vi "VMI Tomography.vi"() -> ()   [LabVIEW 2019]
uses:
  <vilib>/vision/NI_Vision_Development_Module.lvlib
panel:
  in  "CONTROL QWP":refnum<k7>(container)
  in  "Tab Control":enum32{"Setup & Align", "Acquire - Tomography"}(tab)
  out "Counts per Laser Shot :":dbl format="%#.1g"
  in  "Image Size (pixels) :":dbl=400.0
  in  "?":bool
  in  "Acquiring :":bool
  in  "Save?":bool
  in  "Mask Width (pixels) :":dbl
  in  "Mask Centre :":bool
  in  "Threshold Level (%) :":dbl
  in  "Image Centre (x,y) : 2":dbl=223.0
  in  "Image Centre (x,y) :":dbl=312.0
  in  "Symmetrise L/R :":bool
  in  "Symmetrise U/D :":bool
  in  "Centroiding :":bool
  out "Test View":dbl[][](graph)
  out "Integrated Signal Graph":dbl[](graph)
  out "Live Camera View":dbl[][](graph)
  in  "QWP Zero Position :":dbl=174.0
  out "Current Scan :":dbl
  out "Current Angle :":dbl
  out "Current Frame :":i32
  in  "Frames per Scan :":dbl=100.0
  out "Current Image":dbl[][](graph)
  in  "?":refnum<k7>(container)
  in  "Molecule :":string="a_pinene"
  in  "OK Button 2":bool
  in  "HWP Zero Position :":dbl=25.7
  in  "HWP Step Size :":dbl=15.0
  in  "No. of Scans :":dbl=1.0
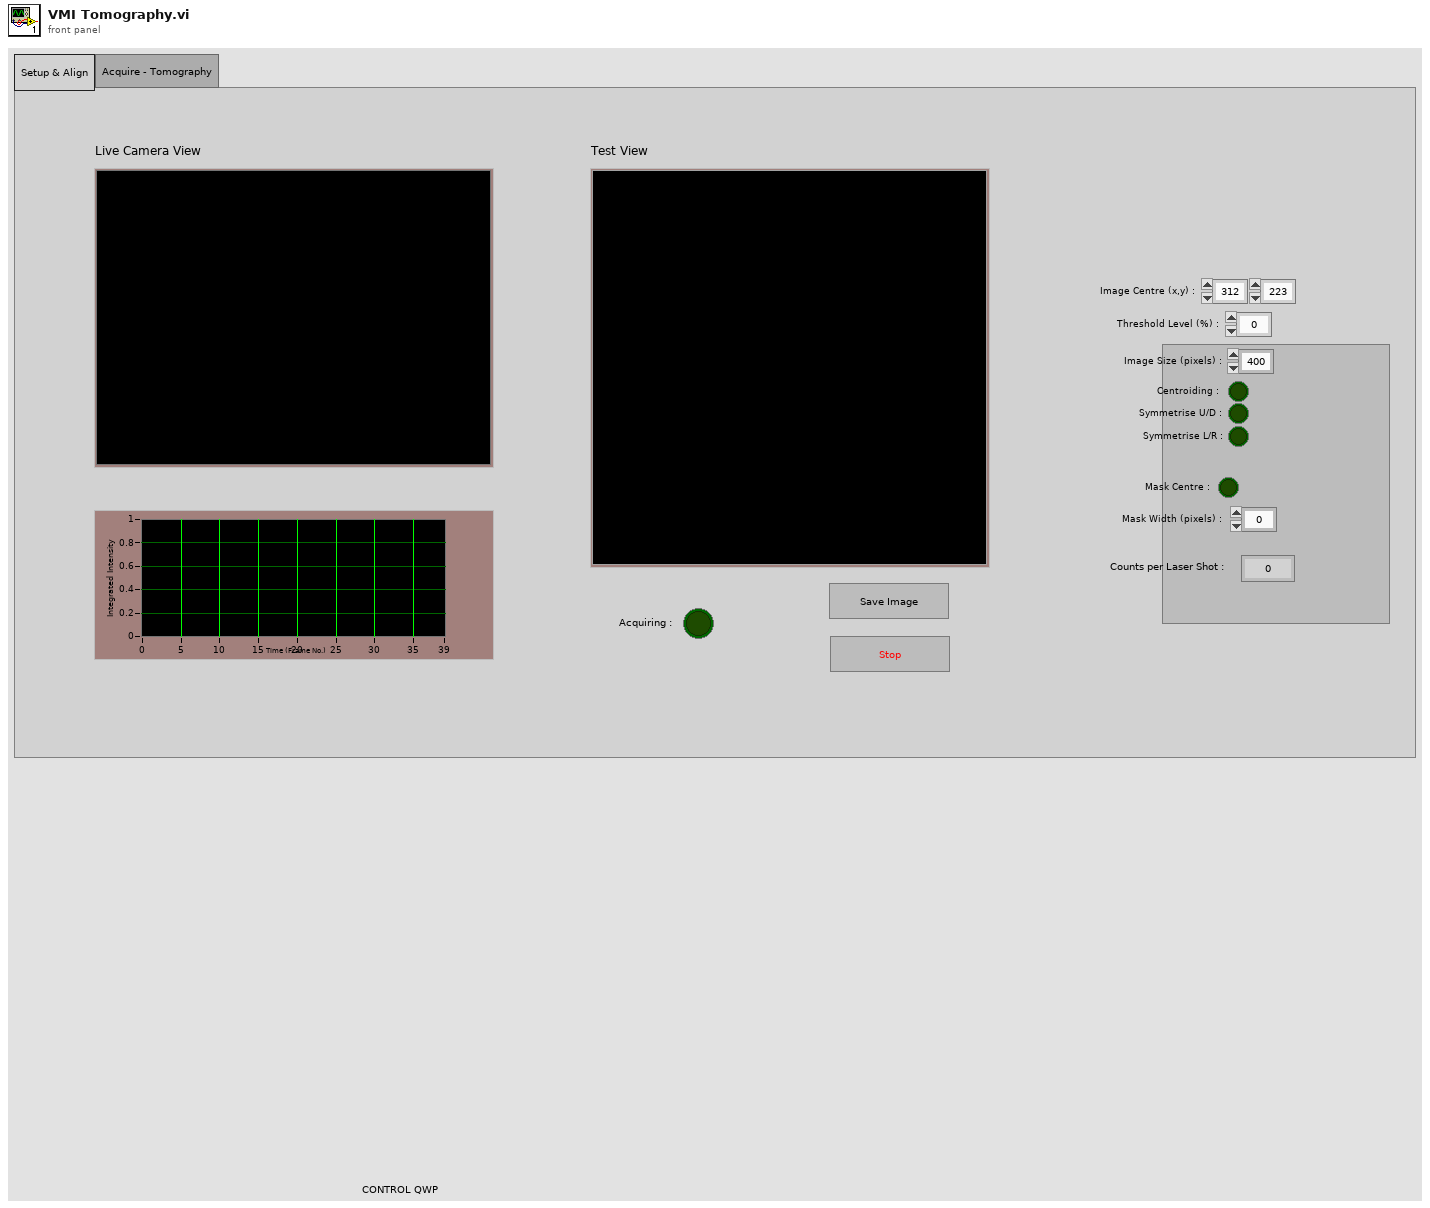
[diagram p1: front panel]
types:
  T1 = typedef "Image Type" = u32
  T2 = typedef "IMAQ Image.ctl" = refnum<image>
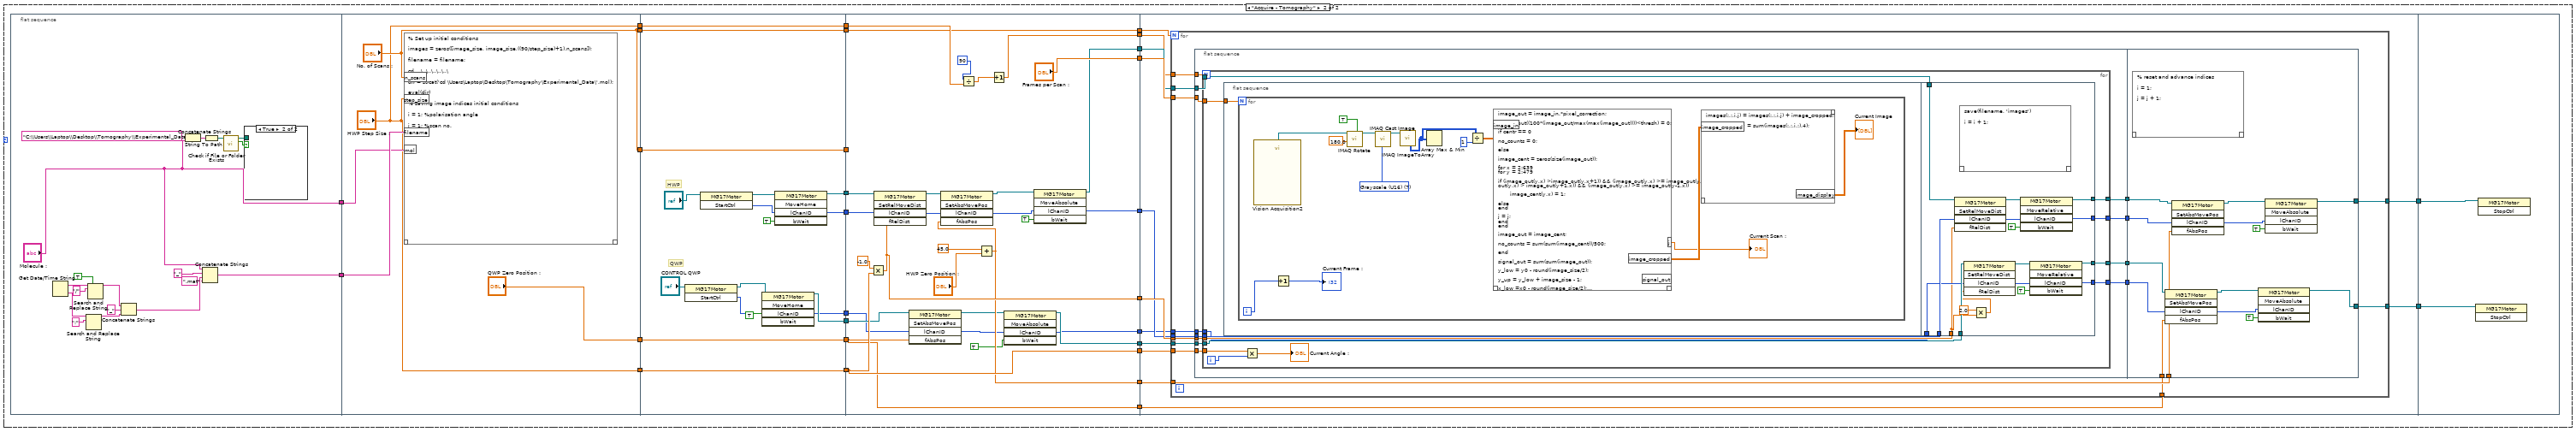
[diagram p3: hidden frame]
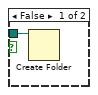
[diagram p4: hidden frame]
diagram:
  n1 = case shown="\"Setup & Align\", Default" "Tab Control" {
    frame "Setup & Align", Default {
      n2 = while {
        i -> [w4]
        stop <- "?" stop-if-true
        n3 = flat-sequence {
          tunnel: [w9] -> w8
          tunnel: w8 -> [w37]
          tunnel: [w36] -> w7
          tunnel: [w35] -> w5
          tunnel: [w31] -> w3
          tunnel: [w18] -> w2
          tunnel: w7 -> [w44]
          tunnel: w5 -> [w40]
          tunnel: w4 -> [_]
          tunnel: w3 -> [w41]
          tunnel: w2 -> [w38]
          frame #0 {
            n4 = script code="% Set up initial variables and define hot pixels\n\npixel_correction = ones(480,640);\n\npixel_correction(445,233) = 0;\npixel_correction(444,232) = 0\npixel_correction(240,208) = 0;\npixel_correction(268,295) = 0;\npixel_correction(440,333) = 0;\npixel_correction(257,482) = 0;\npixel_correction(128,286) = 0;\npixel_correction(208,240) = 0;\npixel_correction(404,604) = 0;\n\npixel_correction(270,304) = 0;\npixel_correction(346,358) = 0;\npixel_correction(220,79) = 0;\npixel_correction(79,218) = 0;\npixel_correction(96,220) = 0;\n\npixel_correction(218,96) = 0;\npixel_correction(268,304) = 0;\npixel_correction(218,79) = 0;\npixel_correction(268,304) = 0;\n\ncd ..\\..\\..\\..\\..\\..\\..\\Users\\Laptop\\Desktop"() -> ()  [unwired: 1 in, 1 out]
          }
          frame #1 {
            w17 = T1 7 items=["Grayscale (U8)", "Grayscale (I16)", "Grayscale (SGL)", "Complex (CSG)", "RGB (U32)", "HSL (U32)", "RGB (U64)", "Grayscale (U16)"] ("Image Type")
            n5 = call "Vision Acquisition"() -> ("Image Out"=w11:T2)  [unwired: 26 in, 1 out]
            n6 = call "IMAQ Rotate"("Maintain Size"=TRUE, "Angle (degrees)"=sgl 180.0, "Image Src"=w11) -> ("Image Dst Out"=w14:T2)  [unwired: 7 in, 1 out]
            n7 = call "IMAQ Cast Image"("Image Type"=w17, "Image Src"=w14) -> ("Image Dst Out"=w16:T2)  [unwired: 8 in, 1 out]
            n8 = call "IMAQ ImageToArray"("Image"=w16) -> ("Image Pixels (U16)"=w15:u16[][])  [unwired: 3 in, 4 out]
            n9 = Array Max & Min(array=w15) -> ()  [unwired: 4 out]
            n10 = Divide(x=w15, y=1) -> (x/y=w9:dbl[][])
          }
          frame #2 {
            n11 = Boolean To (0,1)(Boolean="Mask Centre :") -> (0, 1=w22:i16)
            n12 = Boolean To (0,1)(Boolean="Acquiring :") -> (0, 1=w25:i16)
            n13 = Boolean To (0,1)(Boolean="Symmetrise U/D :") -> (0, 1=w26:i16)
            n14 = Boolean To (0,1)(Boolean="Symmetrise L/R :") -> (0, 1=w29:i16)
            n15 = Boolean To (0,1)(Boolean="Centroiding :") -> (0, 1=w19:i16)
            n16 = script code="image_out = image_in.*pixel_correction;\n\nimage_out((100*(image_out/max(max(image_out))))<thresh) = 0;\n\nif centr == 0\n\nno_counts = 0;\n\nelse\n\nimage_cent = zeros(size(image_out));\n\nfor x = 2:639\nfor y = 2:479\n\nif (image_out(y,x) >image_out(y,x+1)) && (image_out(y,x) >= image_out(y,x-1)) && (image_out(y,x) > image_out(y+1,x)) && (image_out(y,x) >= image_out(y-1,x))\n\n       image_cent(y,x) = 1;\n\nelse\nend\n\nend\nend\n\nimage_out = image_cent;\n\nno_counts = sum(sum(image_cent))/500;\n\nend\n\nsignal_out = sum(sum(image_out));\n\ny_low = y0 - round(image_size/2);\n\ny_up = y_low + image_size - 1;\n\nx_low =x0 - round(image_size/2);\n\nx_up = x_low + image_size - 1;\n\nif acqu == 0\n\n     image_cropped = zeros(image_size);\n\nend\n\nimage_cropped = image_out(y_low:y_up,x_low:x_up) + image_cropped;\n\nif LR == 1\n\n     image_cropped = 0.5*(image_cropped + fliplr(image_cropped));\n\nend\n\nif UD == 1\n\n     image_cropped = 0.5*(image_cropped + flipud(image_cropped));\n\nend\n\nif mask == 1\n\n     x = linspace(-(round(image_size/2)), round(image_size/2), image_size);\n\n     [X, Y] = meshgrid(x,x);\n\n     R = sqrt(X.^2 + Y.^2);\n\n     mask_ = ones(size(R));\n\n     mask_(R<mask_width) = 0;\n\n     image_cropped = image_cropped.*mask_;\n\nend\n\nrange = 1:image_size;\n\ny_int = sum(image_cropped,1);\ny_int = y_int/max(y_int);\n\nx_int = sum(image_cropped,2);\nx_int = x_int/max(x_int);"("image_in"=w37, "image_size"="Image Size (pixels) :", "x0"="Image Centre (x,y) :", "y0"="Image Centre (x,y) : 2", "thresh"="Threshold Level (%) :", "LR"=w29, "UD"=w26, "acqu"=w25, "mask"=w22, "mask_width"="Mask Width (pixels) :", "centr"=w19) -> ("image_out"=w36:dbl[][], "signal_out"=w35:dbl, "image_cropped"=w31:dbl[][], "no_counts"=w18:dbl)  [unwired: 1 in, 4 out]
          }
          frame #3 {
            n17 = feedback #1() -> (w39:dbl[])  [unwired: 1 in]
            n18 = Build Array (concatenate)(w39, w40) -> (w48:dbl[])
            n19 = feedback-in #1(w48) -> ()
            n20 = Array Max & Min(array=w44) -> (max value=w45:dbl)  [unwired: 3 out]
            n21 = Array Max & Min(array=w41) -> (max value=w43:dbl)  [unwired: 3 out]
            n22 = Array Max & Min(array=w48) -> (max value=w47:dbl)  [unwired: 3 out]
            n23 = Divide(x=w44, y=w45) -> (x/y=→"Live Camera View":dbl[][])
            n24 = Divide(x=w41, y=w43) -> (x/y=→"Test View":dbl[][])
            n25 = Divide(x=w48, y=w47) -> (x/y=→"Integrated Signal Graph":dbl[])
            "Counts per Laser Shot :" <- w38
          }
          frame #4 {
            n26 = case shown="True" "Save?" {
              frame False {
              }
              frame True {
                n27 = script code="image = image_cropped;\n\nuisave('image','image.mat')"() -> ()  [unwired: 1 in, 1 out]
              }
            }
          }
        }
      }
    }
    frame "Acquire - Tomography" {
      n28 = flat-sequence {
        tunnel: [w81] -> w73
        tunnel: ["Molecule :"] -> w72
        tunnel: ["No. of Scans :"] -> w76
        tunnel: ["HWP Step Size :"] -> w74
        tunnel: w73 -> [w103]
        tunnel: w72 -> [w102]
        tunnel: ["No. of Scans :"] -> w71
        tunnel: ["HWP Step Size :"] -> w64
        tunnel: ["QWP Zero Position :"] -> w56
        tunnel: [w116] -> w79
        tunnel: [w115] -> w78
        tunnel: [w114] -> w77
        tunnel: w76 -> [w114]
        tunnel: [w113] -> w75
        tunnel: w74 -> [w113]
        tunnel: w71 -> [w112]
        tunnel: [w112] -> w70
        tunnel: [w111] -> w65
        tunnel: w64 -> [w111]
        tunnel: [w106] -> w58
        tunnel: [w105] -> w57
        tunnel: w56 -> [w104]
        tunnel: [w104] -> w55
        tunnel: w79 -> [w149]
        tunnel: w78 -> [w148]
        tunnel: w77 -> [w129]
        tunnel: w75 -> [w131]
        tunnel: w70 -> [_]
        tunnel: ["Frames per Scan :"] -> w69
        tunnel: [w138] -> w68
        tunnel: [w137] -> w67
        tunnel: [w136] -> w66
        tunnel: w65 -> [w135]
        tunnel: [w132] -> w63
        tunnel: [w131] -> w62
        tunnel: [w130] -> w61
        tunnel: [w129] -> w60
        tunnel: w58 -> [w125]
        tunnel: w57 -> [w124]
        tunnel: w55 -> [w121]
        tunnel: [w123] -> w54
        tunnel: [w122] -> w53
        tunnel: [w121] -> w51
        tunnel: w69 -> [w162]
        tunnel: w68 -> [w161]
        tunnel: w67 -> [w160]
        tunnel: w66 -> [w159]
        tunnel: w63 -> [w158]
        tunnel: w62 -> [w157]
        tunnel: w61 -> [w156]
        tunnel: w60 -> [w155]
        tunnel: [w154] -> w59
        tunnel: w54 -> [w153]
        tunnel: w53 -> [w152]
        tunnel: [w151] -> w52
        tunnel: w51 -> [w150]
        tunnel: w59 -> [w251]
        tunnel: w52 -> [w250]
        frame #0 {
          n29 = Get Date/Time String() -> (date string=w92:string, time string=w89:string)  [unwired: 3 in]
          n30 = Search and Replace String(input string=w89, search string=":") -> (result string=w86:string)  [unwired: 6 in, 3 out]
          n31 = Search and Replace String(replace all?=TRUE ("replace all? (F)"), input string=w92, search string="/") -> (result string=w87:string)  [unwired: 5 in, 3 out]
          n32 = Concatenate Strings(w87, "_" ("string"), w86) -> (w83:string)
          n33 = Concatenate Strings("C:\\Users\\Laptop\\Desktop\\Tomography\\Experimental_Data\\", "Molecule :") -> (w93:string)
          n34 = Concatenate Strings("Molecule :", "_" ("string"), w83, ".mat" ("string")) -> (w81:string)
          n35 = String To Path(string=w93) -> (path=w96:path)
          n36 = call <vilib>:"Check if File or Folder Exists.vi"("path"=w96) -> ("file or folder exists?"=w95:bool, "dup path"=w94:path)  [unwired: 8 in, 1 out]
          n37 = case shown="True" w95 {
            tunnel: w94 -> [w98 _]
            frame False {
              n38 = Create Folder(path (use dialog)=w98) -> ()  [unwired: 2 in, 3 out]
            }
            frame True {
            }
          }
        }
        frame #1 {
          n39 = script code="% Set up initial conditions\n\nimages = zeros([image_size, image_size,((90/step_size)+1),n_scans]);\n\nfilename = filename;\n\ncd  ..\\..\\..\\..\\..\\..\\\n\ndir = strcat('cd \\Users\\Laptop\\Desktop\\Tomography\\Experimental_Data\\',mol);\n\neval(dir)\n\n% saving image indices initial conditions\n\ni = 1; %polarisation angle\n\nj = 1; %scan no."("n_scans"="No. of Scans :", "step_size"="HWP Step Size :", "filename"=w103, "mol"=w102) -> ()  [unwired: 1 in, 1 out]
        }
        frame #2 {
          # "QWP"
          # "HWP"
          n40 = invoke class="MG17Motor" method="StartCtrl"(reference="CONTROL QWP") -> (reference out=w108:refnum<k7>, "StartCtrl"=w107:i32)  [unwired: 2 in, 1 out]
          n41 = invoke class="MG17Motor" method="StartCtrl"(reference="?") -> (reference out=w119:refnum<k7>, "StartCtrl"=w118:i32)  [unwired: 2 in, 1 out]
          n42 = invoke class="MG17Motor" method="MoveHome"(reference=w108, "lChanID"=w107, "bWait"=TRUE) -> (reference out=w106:refnum<k7>, "lChanID"=w105:i32)  [unwired: 2 in, 3 out]
          n43 = invoke class="MG17Motor" method="MoveHome"(reference=w119, "lChanID"=w118, "bWait"=TRUE) -> (reference out=w116:refnum<k7>, "lChanID"=w115:i32)  [unwired: 2 in, 3 out]
        }
        frame #3 {
          n44 = Multiply(x=-1.0, y=w131) -> (x*y=w138:dbl)
          n45 = invoke class="MG17Motor" method="SetRelMoveDist"(reference=w149, "lChanID"=w148, "fRelDist"=w138) -> (reference out=w147:refnum<k7>, "lChanID"=w146:i32)  [unwired: 2 in, 3 out]
          n46 = invoke class="MG17Motor" method="SetAbsMovePos"(reference=w125, "lChanID"=w124, "fAbsPos"=w121) -> (reference out=w128:refnum<k7>, "lChanID"=w127:i32)  [unwired: 2 in, 3 out]
          n47 = Divide(x=90, y=w135) -> (x/y=w133:dbl)
          n48 = Add(x=45.0, y="HWP Zero Position :") -> (x+y=w130:dbl)
          n49 = invoke class="MG17Motor" method="SetAbsMovePos"(reference=w147, "lChanID"=w146, "fAbsPos"=w130) -> (reference out=w143:refnum<k7>, "lChanID"=w142:i32)  [unwired: 2 in, 3 out]
          n50 = Increment(x=w133) -> (x+1=w132:dbl)
          n51 = invoke class="MG17Motor" method="MoveAbsolute"(reference=w128, "lChanID"=w127, "bWait"=TRUE) -> (reference out=w123:refnum<k7>, "lChanID"=w122:i32)  [unwired: 2 in, 3 out]
          n52 = invoke class="MG17Motor" method="MoveAbsolute"(reference=w143, "lChanID"=w142, "bWait"=TRUE) -> (reference out=w136:refnum<k7>, "lChanID"=w137:i32)  [unwired: 2 in, 3 out]
        }
        frame #4 {
          n53 = for {
            N: w155 -> [_]
            tunnel: w162 -> [w178]
            tunnel: w161 -> [w177]
            tunnel: w160 -> [w176]
            tunnel: w159 -> [w175]
            tunnel: w158 -> [w174]
            tunnel: w157 -> [w173]
            tunnel: w156 -> [w170]
            tunnel: [w169] -> w154
            tunnel: w153 -> [w168]
            tunnel: w152 -> [w167]
            tunnel: [w164] -> w151
            tunnel: w150 -> [w163]
            n54 = flat-sequence {
              tunnel: w178 -> [w190]
              tunnel: w177 -> [w189]
              tunnel: w176 -> [w188]
              tunnel: w175 -> [w187]
              tunnel: w174 -> [w186]
              tunnel: w173 -> [w185]
              tunnel: [w184] -> w172
              tunnel: [w183] -> w171
              tunnel: w168 -> [w182]
              tunnel: w167 -> [w181]
              tunnel: [w180] -> w166
              tunnel: [w179] -> w165
              tunnel: w172 -> [w246]
              tunnel: w171 -> [w245]
              tunnel: w170 -> [w244]
              tunnel: [w243] -> w169
              tunnel: w166 -> [w239]
              tunnel: w165 -> [w238]
              tunnel: [w237] -> w164
              tunnel: w163 -> [w236]
              frame #0 {
                n55 = for {
                  N: w186 -> [_]
                  tunnel: w190 -> [w203]
                  tunnel: w189 -> [w202]
                  tunnel: w188 -> [w201]
                  tunnel: w187 -> [w200]
                  tunnel: w185 -> [w198]
                  tunnel: [w196] -> w184
                  tunnel: [w195] -> w183
                  tunnel: w182 -> [w194]
                  tunnel: w181 -> [w193]
                  tunnel: [w192] -> w180
                  tunnel: [w191] -> w179
                  i -> [w199]
                  n56 = flat-sequence {
                    tunnel: w203 -> [w204]
                    tunnel: w202 -> [w223]
                    tunnel: w201 -> [w235]
                    tunnel: w200 -> [w232]
                    tunnel: [w230] -> w196
                    tunnel: [w229] -> w195
                    tunnel: w194 -> [w225]
                    tunnel: w193 -> [w224]
                    tunnel: [w220] -> w192
                    tunnel: [w219] -> w191
                    frame #0 {
                      n57 = for {
                        N: w204 -> [_]
                        i -> [w207]
                        w218 = T1 7 items=["Grayscale (U8)", "Grayscale (I16)", "Grayscale (SGL)", "Complex (CSG)", "RGB (U32)", "HSL (U32)", "RGB (U64)", "Grayscale (U16)"] ("Image Type")
                        n58 = call "Vision Acquisition2"() -> ("Image Out"=w212:T2)  [unwired: 26 in, 1 out]
                        n59 = Increment(x=w207) -> (x+1=→"Current Frame :":i32)
                        n60 = call "IMAQ Rotate"("Maintain Size"=TRUE, "Angle (degrees)"=sgl 180.0, "Image Src"=w212) -> ("Image Dst Out"=w215:T2)  [unwired: 7 in, 1 out]
                        n61 = call "IMAQ Cast Image"("Image Type"=w218, "Image Src"=w215) -> ("Image Dst Out"=w217:T2)  [unwired: 8 in, 1 out]
                        n62 = call "IMAQ ImageToArray"("Image"=w217) -> ("Image Pixels (U16)"=w216:u16[][])  [unwired: 3 in, 4 out]
                        n63 = Array Max & Min(array=w216) -> ()  [unwired: 4 out]
                        n64 = Divide(x=w216, y=1) -> (x/y=w210:dbl[][])
                        n65 = script code="image_out = image_in.*pixel_correction;\n\nimage_out((100*(image_out/max(max(image_out))))<thresh) = 0;\n\nif centr == 0\n\nno_counts = 0;\n\nelse\n\nimage_cent = zeros(size(image_out));\n\nfor x = 2:639\nfor y = 2:479\n\nif (image_out(y,x) >image_out(y,x+1)) && (image_out(y,x) >= image_out(y,x-1)) && (image_out(y,x) > image_out(y+1,x)) && (image_out(y,x) >= image_out(y-1,x))\n\n       image_cent(y,x) = 1;\n\nelse\nend\n\nj = j;\nend\nend\n\nimage_out = image_cent;\n\nno_counts = sum(sum(image_cent))/500;\n\nend\n\nsignal_out = sum(sum(image_out));\n\ny_low = y0 - round(image_size/2);\n\ny_up = y_low + image_size - 1;\n\nx_low =x0 - round(image_size/2);\n\nx_up = x_low + image_size - 1;\n\nif acqu == 0\n\n     image_cropped = zeros(image_size);\n\nend\n\nimage_cropped = image_out(y_low:y_up,x_low:x_up) + image_cropped;\n\nif LR == 1\n\n     image_cropped = 0.5*(image_cropped + fliplr(image_cropped));\n\nend\n\nif UD == 1\n\n     image_cropped = 0.5*(image_cropped + flipud(image_cropped));\n\nend\n\nif mask == 1\n\n     x = linspace(-(round(image_size/2)), round(image_size/2), image_size);\n\n     [X, Y] = meshgrid(x,x);\n\n     R = sqrt(X.^2 + Y.^2);\n\n     mask_ = ones(size(R));\n\n     mask_(R<mask_width) = 0;\n\n     image_cropped = image_cropped.*mask_;\n\nend\n\nrange = 1:image_size;\n\ny_int = sum(image_cropped,1);\ny_int = y_int/max(y_int);\n\nx_int = sum(image_cropped,2);\nx_int = x_int/max(x_int);"("image_in"=w210) -> ("image_cropped"=w209:dbl[][], "j"=→"Current Scan :":dbl)  [unwired: 1 in, 2 out]
                        n66 = script code="images(:,:,i,j) = images(:,:,i,j) + image_cropped;\n\nimage_display = sum(images(:,:,i,:),4);"("image_cropped"=w209) -> ("image_display"=→"Current Image":dbl[][])  [unwired: 1 in, 1 out]
                      }
                    }
                    frame #1 {
                      n67 = invoke class="MG17Motor" method="SetRelMoveDist"(reference=w232, "lChanID"=w235, "fRelDist"=w223) -> (reference out=w231:refnum<k7>, "lChanID"=w234:i32)  [unwired: 2 in, 3 out]
                      n68 = script code="save(filename, 'images')\n\ni = i + 1;"() -> ()  [unwired: 1 in, 1 out]
                      n69 = Multiply(x=2.0, y=w223) -> (x*y=w221:dbl)
                      n70 = invoke class="MG17Motor" method="SetRelMoveDist"(reference=w225, "lChanID"=w224, "fRelDist"=w221) -> (reference out=w226:refnum<k7>, "lChanID"=w228:i32)  [unwired: 2 in, 3 out]
                      n71 = invoke class="MG17Motor" method="MoveRelative"(reference=w231, "lChanID"=w234, "bWait"=TRUE) -> (reference out=w229:refnum<k7>, "lChanID"=w230:i32)  [unwired: 2 in, 3 out]
                      n72 = invoke class="MG17Motor" method="MoveRelative"(reference=w226, "lChanID"=w228, "bWait"=TRUE) -> (reference out=w220:refnum<k7>, "lChanID"=w219:i32)  [unwired: 2 in, 3 out]
                    }
                  }
                  n73 = Multiply(x=w198, y=w199) -> (x*y=→"Current Angle :":dbl)
                }
              }
              frame #1 {
                n74 = script code="% reset and advance indices\n\ni = 1;\n\nj = j + 1;"() -> ()  [unwired: 1 in, 1 out]
                n75 = invoke class="MG17Motor" method="SetAbsMovePos"(reference=w239, "lChanID"=w238, "fAbsPos"=w236) -> (reference out=w242:refnum<k7>, "lChanID"=w241:i32)  [unwired: 2 in, 3 out]
                n76 = invoke class="MG17Motor" method="SetAbsMovePos"(reference=w245, "lChanID"=w246, "fAbsPos"=w244) -> (reference out=w249:refnum<k7>, "lChanID"=w248:i32)  [unwired: 2 in, 3 out]
                n77 = invoke class="MG17Motor" method="MoveAbsolute"(reference=w242, "lChanID"=w241, "bWait"=TRUE) -> (reference out=w237:refnum<k7>)  [unwired: 2 in, 4 out]
                n78 = invoke class="MG17Motor" method="MoveAbsolute"(reference=w249, "lChanID"=w248, "bWait"=TRUE) -> (reference out=w243:refnum<k7>)  [unwired: 2 in, 4 out]
              }
            }
          }
        }
        frame #5 {
          n79 = invoke class="MG17Motor" method="StopCtrl"(reference=w250) -> ()  [unwired: 2 in, 3 out]
          n80 = invoke class="MG17Motor" method="StopCtrl"(reference=w251) -> ()  [unwired: 2 in, 3 out]
        }
      }
    }
  }
